vi "Update RPC Template Accessor.vi"(8 "error in (no error)":errorcluster, 10 "Accessor Name":string, 11 "Server Library (Library Item) in":refnum<vi>) -> (0 "error out":errorcluster, 3 "Server Library (Library Item) out":refnum<vi>)   [LabVIEW 2019, in "gRPC Scripting Tools.lvlib"]
uses:
  gRPC Scripting Tools.lvlib
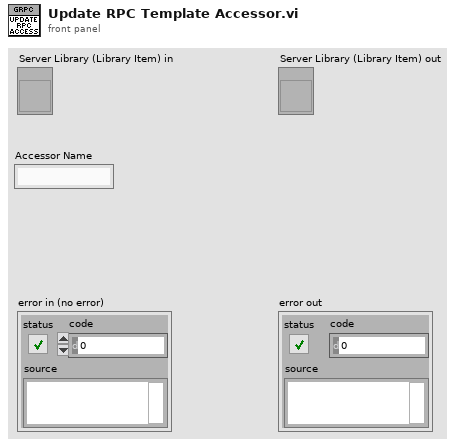
[diagram p1: front panel]
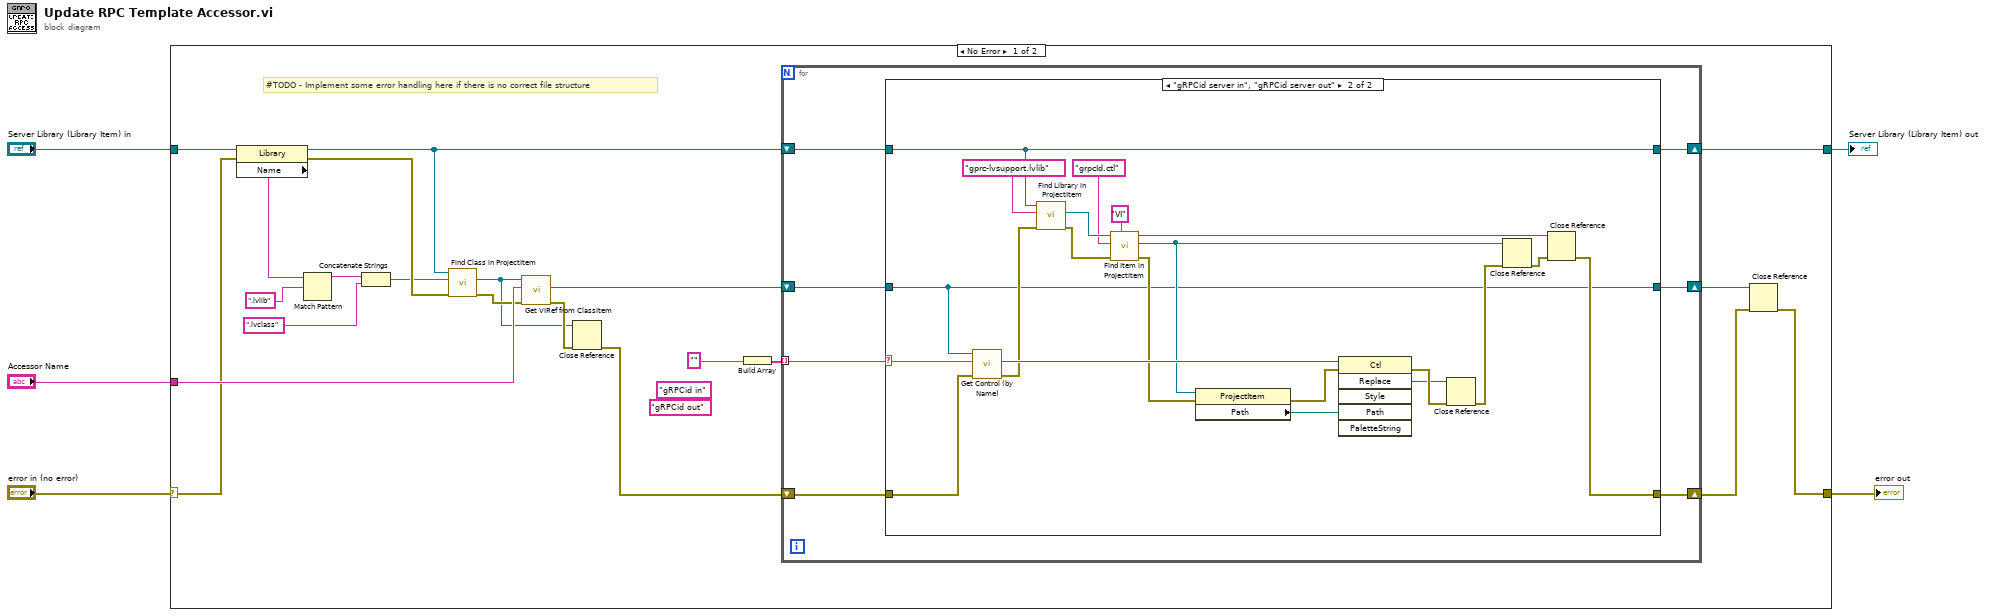
[diagram p0: block diagram]
diagram:
  n1 = case shown="No Error" "error in (no error)" {
    selector: "error in (no error)" -> [w11 w58]
    tunnel: [w26 w59] -> w5
    tunnel: "Server Library (Library Item) in" -> [w13 w59]
    tunnel: "Accessor Name" -> [w23 _]
    tunnel: [w20 w58] -> w2
    frame No Error {
      (unwired) "gRPCid out" ("Item Name")
      (unwired) "gRPCid in" ("Item Name")
      # "#TODO - Implement some error handling here if there is no correct file structure"
      n2 = property class="Library"(reference=w13, error in=w11) -> (reference out=w12:refnum<vi>, error out=w19:errorcluster, "Name"=w16:string)
      n3 = Match Pattern(string=w16, regular expression=".lvlib") -> (before substring=w17:string)  [unwired: 1 in, 3 out]
      n4 = Concatenate Strings(w17, ".lvclass" ("string")) -> (w18:string)
      n5 = call "Find Class in ProjectItem.vi"("error in (no error)"=w19, "Class Name"=w18, "ProjectItem in"=w12) -> ("error out"=w10:errorcluster, "LVClass out"=w8:refnum<vi>)  [unwired: 5 in, 2 out]
      n6 = call "Get VIRef from ClassItem.vi"("error in (no error)"=w10, "Item Name"=w23, "LVClassLibrary in"=w8) -> ("error out"=w9:errorcluster, "VIref out"=w24:refnum<vi>)  [unwired: 5 in, 2 out]
      n7 = Close Reference(reference=w8, error in (no error)=w9) -> (error out=w7:errorcluster)
      n8 = Build Array("") -> (w25:string[])
      n9 = for {
        tunnel: w25 -> [w33] mode=indexing
        shift-right: [w31] -> w26
        shift-left: w12 -> [w32]
        shift-right: [w28] -> w22
        shift-left: w7 -> [w29]
        shift-right: [w27] -> w21
        shift-left: w24 -> [w30]
        n10 = case shown="\"gRPCid server in\", \"gRPCid server out\"" w33 {
          selector: w33 -> [_ w40]
          tunnel: w32 -> [w36 w41]
          tunnel: [w36 w41] -> w31
          tunnel: w30 -> [w35 w37]
          tunnel: w29 -> [w34 w39]
          tunnel: [w34 w38] -> w28
          tunnel: [w35 w37] -> w27
          frame "False", Default {
          }
          frame "gRPCid server in", "gRPCid server out" {
            n11 = call "Get Control (by Name).vi"("error in (no error)"=w39, "Control Label"=w40, "Owner VI in"=w37) -> ("error out"=w51:errorcluster, "Control Refnum"=w53:refnum<vi>)  [unwired: 5 in, 2 out]
            n12 = call "Find Library in ProjectItem.vi"("error in (no error)"=w51, "Library Name"="gprc-lvsupport.lvlib", "ProjectItem in"=w41) -> ("error out"=w50:errorcluster, "Library out"=w56:refnum<vi>)  [unwired: 5 in, 2 out]
            n13 = call "Find Item in ProjectItem.vi"("Item Type"="VI", "error in (no error)"=w50, "Name"="grpcId.ctl", "ProjectItem in"=w56) -> ("error out"=w49:errorcluster, "Item Refnum out"=w44:refnum<vi>, "ProjectItem out"=w42:refnum<vi>)  [unwired: 4 in, 1 out]
            n14 = property class="ProjectItem"(reference=w44, error in=w49) -> (error out=w46:errorcluster, "Path"=w52:path)  [unwired: 1 out]
            n15 = invoke class="Ctl" method="Replace"(reference=w53, error in=w46, "Path"=w52) -> (error out=w48:errorcluster, "Replace"=w47:refnum<vi>)  [unwired: 3 in, 4 out]
            n16 = Close Reference(reference=w47, error in (no error)=w48) -> (error out=w45:errorcluster)
            n17 = Close Reference(reference=w44, error in (no error)=w45) -> (error out=w43:errorcluster)
            n18 = Close Reference(reference=w42, error in (no error)=w43) -> (error out=w38:errorcluster)
          }
        }
      }
      n19 = Close Reference(reference=w21, error in (no error)=w22) -> (error out=w20:errorcluster)
    }
    frame Error {
    }
  }
  "Server Library (Library Item) out" <- w5
  "error out" <- w2
